vi "Add Block Diagram Content.vi"(8 "error in (no error)":errorcluster, 9 "Term Refnums":refnum<vi>[](array[refnum]), 10 "ModuleLoop":T1, 11 "EST Digital Event in":refnum<class "Digital Event.lvclass">) -> (0 "error out":errorcluster, 3 "EST Digital Event out":refnum<class "Digital Event.lvclass">)   [LabVIEW 2026, in "Digital Event.lvclass"]
uses:
  Digital Event.lvclass
  C:/Projects/VeriStand-FPGA-Generation-Wizard/Source/Classes/Signal/Signal/Signal.lvclass
  VI/VI/Module.Refs.ctl
  <vilib>/Utility/miscctls.llb/LVPointTypeDef.ctl
  <vilib>/_script/New VI Object TypeDefs/NewVIObject_LVRelativePositionTypeDef.ctl
  <vilib>/_script/New VI Object TypeDefs/NewVIObject_LVRelativeDirectionTypeDef.ctl
  <vilib>/Utility/miscctls.llb/LVPoint32TypeDef.ctl
  Read Events.vi
  Signal/Read IP Core Path.vi
  Signal/Read Signal Name.vi
  Read Capture Path.vi
  VI/VI/VI.lvclass
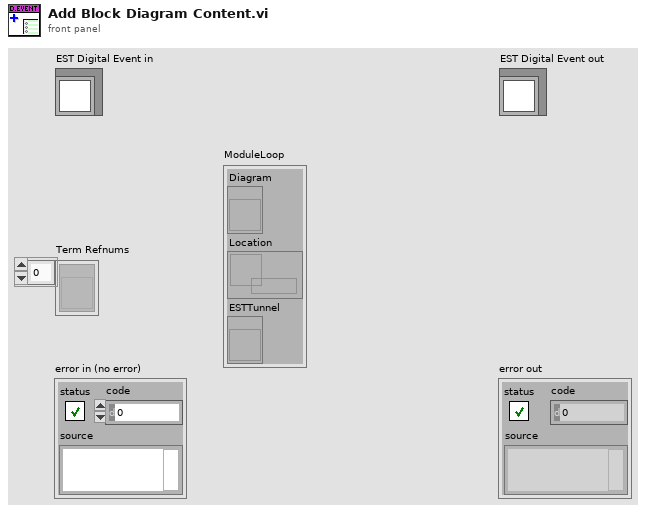
[diagram p1: front panel]
types:
  T1 = typedef "VI.lvclass/Module.Refs.ctl" = cluster{"Diagram":refnum<vi>, "Location":refnum<data-value>, "ESTTunnel":refnum<vi>}
  T2 = typedef "NewVIObject_LVRelativePositionTypeDef.ctl" = cluster{"Refnum":refnum<vi>, "Relative Direction":T3, "Point32":T4}
  T3 = typedef "NewVIObject_LVRelativeDirectionTypeDef.ctl" = enum32{"Right", "Left", "Top", "Bottom", "Top Right", "Top Left", "Bottom Right", "Bottom Left"}
  T4 = typedef "LVPoint32TypeDef.ctl" = cluster{"Horizontal":i32, "Vertical":i32}
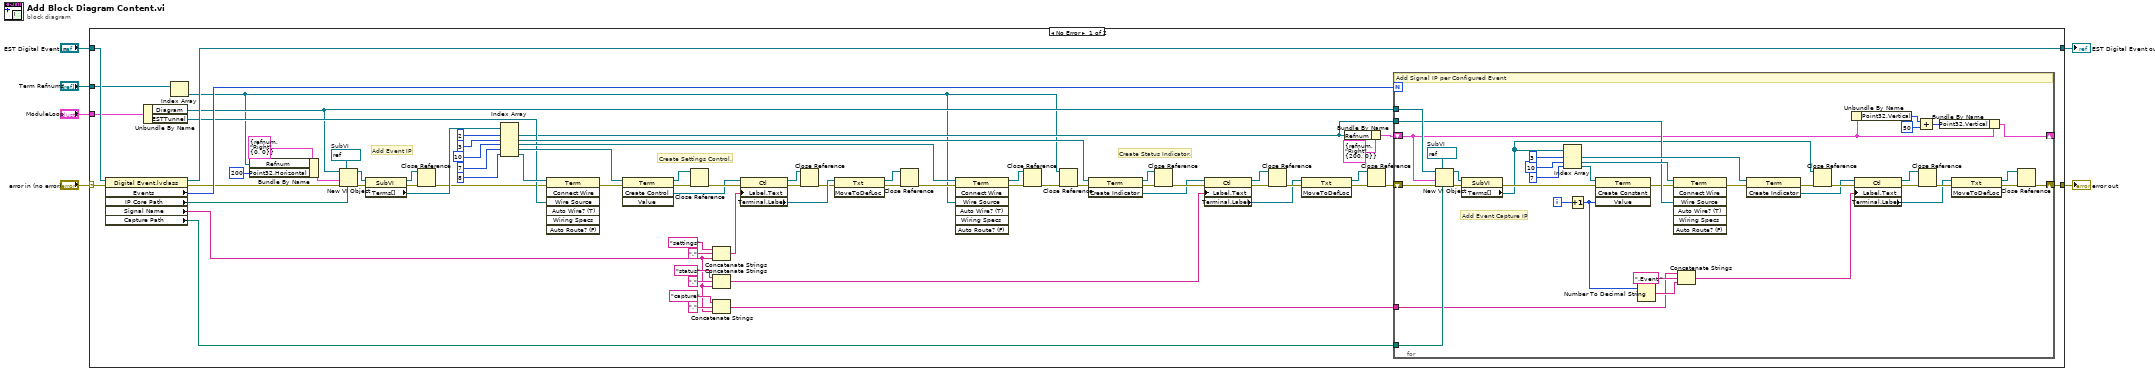
[diagram p0: block diagram]
diagram:
  n1 = case shown="No Error" "error in (no error)" {
    selector: "error in (no error)" -> [w15 w118]
    tunnel: "EST Digital Event in" -> [w33 w117]
    tunnel: [w30 w118] -> w5
    tunnel: [w29 w117] -> w4
    tunnel: "ModuleLoop" -> [w28 _]
    tunnel: "Term Refnums" -> [w24 _]
    frame No Error {
      w59 = refnum<vi> refnum  # SubVI
      # "Create Status Indicator."
      # "Create Settings Control."
      # "Add Event IP"
      n2 = property class="Digital Event.lvclass"(reference=w33, error in=w15) -> (reference out=w29:refnum<class "Digital Event.lvclass">, error out=w21:errorcluster, "Events"=w32:u32, "IP Core Path"=w16:path, "Signal Name"=w8:string, "Capture Path"=w31:path)
      n3 = Unbundle By Name(w28) -> ("Diagram"=w26:refnum<vi>, "ESTTunnel"=w27:refnum<vi>)
      n4 = Index Array(array=w24) -> (element=w7:refnum<vi>)  [unwired: 1 in]
      n5 = Bundle By Name(cluster=T2 {"Refnum"=refnum, "Relative Direction"=enum."Right", "Point32"={"Horizontal"=0, "Vertical"=0}} ("Relative Position"), "Refnum"=w7, "Point32.Horizontal"=200) -> (w22:T2)
      n6 = New VI Object(vi object class=w59, owner refnum=w26, position/next to=w22, 6:w16, 8:w21) -> (object refnum=w61:refnum<vi>, 0:w62:errorcluster)  [unwired: 3 in]
      n7 = property class="SubVI"(reference=w61, error in=w62) -> (reference out=w14:refnum<vi>, error out=w13:errorcluster, "Terms[]"=w60:refnum<vi>[])
      n8 = Close Reference(reference=w14, error in (no error)=w13) -> (error out=w12:errorcluster)
      n9 = Index Array(array=w60, index #1=2 ("index"), index #2=3 ("index"), index #3=10 ("index"), index #4=7 ("index"), index #5=8 ("index")) -> (element #1=w19:refnum<vi>, element #2=w40:refnum<vi>, element #3=w41:refnum<vi>, element #4=w42:refnum<vi>, element #5=w35:refnum<vi>)
      n10 = invoke class="Term" method="Connect Wire"(reference=w35, error in=w12, "Wire Source"=w27) -> (error out=w34:errorcluster)  [unwired: 4 in, 6 out]
      n11 = invoke class="Term" method="Create Control"(reference=w42, error in=w34) -> (reference out=w68:refnum<vi>, error out=w67:errorcluster, "Create Control"=w58:refnum<vi>)  [unwired: 2 in, 1 out]
      n12 = Close Reference(reference=w68, error in (no error)=w67) -> (error out=w69:errorcluster)
      n13 = Concatenate Strings("settings" ("string"), "." ("string"), w8) -> (w63:string)
      n14 = Concatenate Strings("status" ("string"), "." ("string"), w8) -> (w39:string)
      n15 = Concatenate Strings("capture" ("string"), "." ("string"), w8) -> (w37:string)
      n16 = property class="Ctl"(reference=w58, error in=w69, "Label.Text"=w63) -> (reference out=w57:refnum<vi>, error out=w55:errorcluster, "Terminal.Label"=w56:refnum<vi>)
      n17 = Close Reference(reference=w57, error in (no error)=w55) -> (error out=w54:errorcluster)
      n18 = invoke class="Txt" method="MoveToDefLoc"(reference=w56, error in=w54) -> (reference out=w52:refnum<vi>, error out=w53:errorcluster)  [unwired: 1 in, 1 out]
      n19 = Close Reference(reference=w52, error in (no error)=w53) -> (error out=w51:errorcluster)
      n20 = invoke class="Term" method="Connect Wire"(reference=w41, error in=w51, "Wire Source"=w7) -> (reference out=w71:refnum<vi>, error out=w70:errorcluster)  [unwired: 4 in, 5 out]
      n21 = Close Reference(reference=w71, error in (no error)=w70) -> (error out=w72:errorcluster)
      n22 = Close Reference(reference=w7, error in (no error)=w72) -> (error out=w73:errorcluster)
      n23 = invoke class="Term" method="Create Indicator"(reference=w40, error in=w73) -> (reference out=w76:refnum<vi>, error out=w77:errorcluster, "Create Indicator"=w65:refnum<vi>)  [unwired: 1 in]
      n24 = Close Reference(reference=w76, error in (no error)=w77) -> (error out=w78:errorcluster)
      n25 = property class="Ctl"(reference=w65, error in=w78, "Label.Text"=w39) -> (reference out=w74:refnum<vi>, error out=w75:errorcluster, "Terminal.Label"=w48:refnum<vi>)
      n26 = Close Reference(reference=w74, error in (no error)=w75) -> (error out=w49:errorcluster)
      n27 = invoke class="Txt" method="MoveToDefLoc"(reference=w48, error in=w49) -> (reference out=w47:refnum<vi>, error out=w50:errorcluster)  [unwired: 1 in, 1 out]
      n28 = Bundle By Name(cluster=T2 {"Refnum"=refnum, "Relative Direction"=enum."Right", "Point32"={"Horizontal"=200, "Vertical"=0}} ("Relative Position"), "Refnum"=w19) -> (w18:T2)
      n29 = Close Reference(reference=w47, error in (no error)=w50) -> (error out=w17:errorcluster)
      n30 = for {
        N: w32 -> [_]
        shift-right: [w98] -> w30
        shift-left: w17 -> [w92]
        tunnel: w26 -> [w113]
        tunnel: w31 -> [w112]
        tunnel: w37 -> [w80]
        tunnel: w19 -> [w93]
        shift-right: [w87] -> _
        shift-left: w18 -> [w91]
        i -> [w95]
        w114 = refnum<vi> refnum  # SubVI
        # "Add Event Capture IP"
        # "Add Signal IP per Configured Event"
        n31 = New VI Object(vi object class=w114, owner refnum=w113, position/next to=w91, 6:w112, 8:w92) -> (object refnum=w115:refnum<vi>, 0:w116:errorcluster)  [unwired: 3 in]
        n32 = property class="SubVI"(reference=w115, error in=w116) -> (error out=w96:errorcluster, "Terms[]"=w84:refnum<vi>[])  [unwired: 1 out]
        n33 = Index Array(array=w84, index #1=3 ("index"), index #2=10 ("index"), index #3=7 ("index")) -> (element #1=w99:refnum<vi>, element #2=w94:refnum<vi>, element #3=w97:refnum<vi>)
        n34 = Increment(x=w95) -> (x+1=w82:i32)
        n35 = invoke class="Term" method="Create Constant"(reference=w97, error in=w96, "Value"=w82) -> (error out=w85:errorcluster)  [unwired: 1 in, 3 out]
        n36 = Number To Decimal String(number=w82) -> (decimal integer string=w81:string)  [unwired: 1 in]
        n37 = invoke class="Term" method="Connect Wire"(reference=w94, error in=w85, "Wire Source"=w93) -> (error out=w86:errorcluster)  [unwired: 4 in, 6 out]
        n38 = Concatenate Strings(w80, ".Event " ("string"), w81) -> (w79:string)
        n39 = invoke class="Term" method="Create Indicator"(reference=w99, error in=w86) -> (error out=w107:errorcluster, "Create Indicator"=w104:refnum<vi>)  [unwired: 1 in, 1 out]
        n40 = Close Reference(reference=w84, error in (no error)=w107) -> (error out=w108:errorcluster)
        n41 = Unbundle By Name(w91) -> ("Point32.Vertical"=w90:i32)
        n42 = property class="Ctl"(reference=w104, error in=w108, "Label.Text"=w79) -> (reference out=w105:refnum<vi>, error out=w106:errorcluster, "Terminal.Label"=w101:refnum<vi>)
        n43 = Add(x=w90, y=50) -> (x+y=w88:i32)
        n44 = Close Reference(reference=w105, error in (no error)=w106) -> (error out=w102:errorcluster)
        n45 = Bundle By Name(cluster=w91, "Point32.Vertical"=w88) -> (w87:T2)
        n46 = invoke class="Txt" method="MoveToDefLoc"(reference=w101, error in=w102) -> (reference out=w100:refnum<vi>, error out=w103:errorcluster)  [unwired: 1 in, 1 out]
        n47 = Close Reference(reference=w100, error in (no error)=w103) -> (error out=w98:errorcluster)
      }
    }
    frame Error {
    }
  }
  "error out" <- w5
  "EST Digital Event out" <- w4
